vi "Post-Install Custom Action.vi"(10 "Variant":variant) -> (0 "error out":errorcluster)   [LabVIEW 2013]
uses:
  <vilib>/Utility/traverseref.llb/TRef TravTarget.ctl
  <vilib>/Utility/traverseref.llb/VI Scripting - Traverse.lvlib
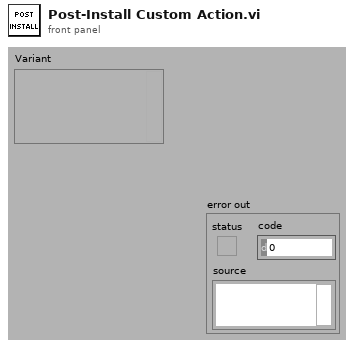
[diagram p1: front panel]
types:
  T1 = typedef "TRef TravTarget.ctl" = enum16{"FP", "BD", "Other"}
  T2 = enum32{"invalid VI type", "Standard VI", "Control VI", "Global VI", "Polymorphic VI", "Configuration VI", "SubSystem", "Facade VI", "Method VI", "Statechart Diagram VI"}
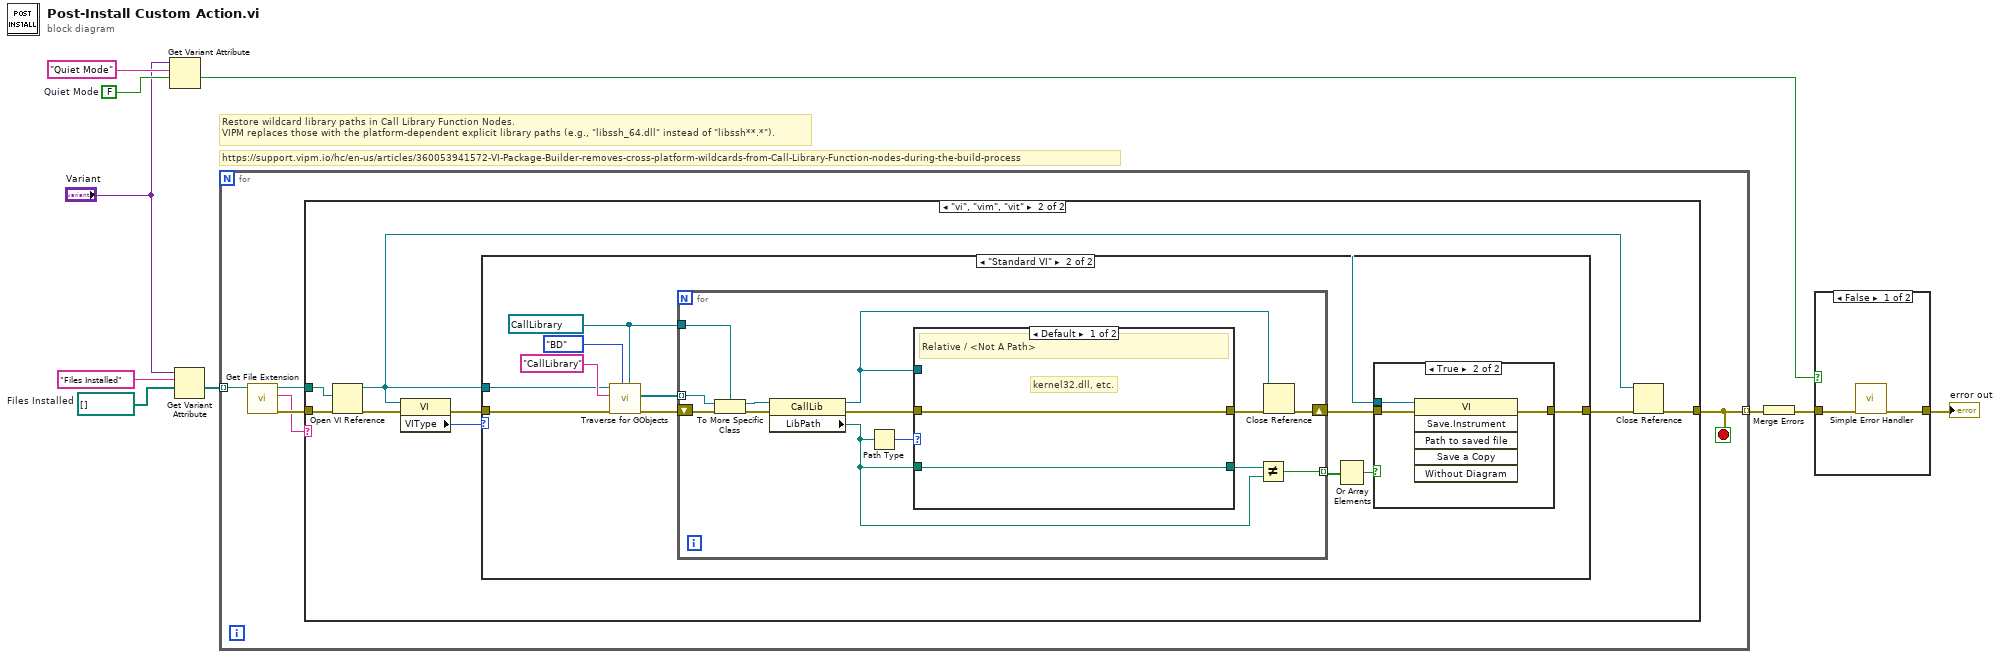
[diagram p0: block diagram]
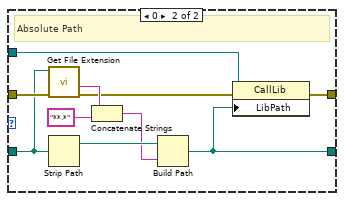
[diagram p6: hidden frame]
diagram:
  w5 = FALSE  # Quiet Mode
  w9 = path[] []  # Files Installed
  # "Restore wildcard library paths in Call Library Function Nodes.\nVIPM replaces those with the platform-dependent explicit library paths (e.g., \"libssh_64.dll\" instead of \"libssh**.*\")."
  # "https://support.vipm.io/hc/en-us/articles/360053941572-VI-Package-Builder-removes-cross-platform-wildcards-from-Call-Library-Function-nodes-during-the-build-process"
  n1 = Get Variant Attribute(Variant="Variant", name="Quiet Mode", default value (empty Variant)=w5) -> (value=w1:bool)  [unwired: 1 in, 3 out]
  n2 = Get Variant Attribute(Variant="Variant", name="Files Installed", default value (empty Variant)=w9) -> (value=w8:path[])  [unwired: 1 in, 3 out]
  n3 = for {
    tunnel: w8 -> [w15] mode=indexing
    tunnel: [w11] -> w7 mode=indexing
    stop <- w11 stop-if-true
    n4 = call <vilib>:"Get File Extension.vi"("file"=w15) -> ("error out"=w13:errorcluster, "lowercase file extension"=w12:string, "dup file"=w14:path)  [unwired: 7 in, 1 out]
    n5 = case shown="\"vi\", \"vim\", \"vit\"" w12 {
      tunnel: w14 -> [_ w24]
      tunnel: [w16 w22] -> w11
      tunnel: w13 -> [w16 w21]
      frame Default {
      }
      frame "vi", "vim", "vit" {
        n6 = Open VI Reference(vi path=w24, error in (no error)=w21) -> (vi reference=w18:refnum<vi>, error out=w20:errorcluster)  [unwired: 4 in]
        n7 = property class="VI"(reference=w18, error in=w20) -> (error out=w19:errorcluster, "VIType"=w17:T2)  [unwired: 1 out]
        n8 = case shown="\"Standard VI\"" w17 {
          tunnel: [w25 w28] -> w23
          tunnel: w19 -> [w25 w27]
          tunnel: w18 -> [_ w26]
          frame Default {
            # "Polimorphic VIs, etc."
          }
          frame "Standard VI" {
            w32 = refnum<vi> refnum ("Other Refnum")
            n9 = call <vilib>:"Traverse for GObjects.vi"("Other Refnum"=w32, "Traverse Target"=TRef_TravTarget."BD", "error in (no error)"=w27, "Class Name"="CallLibrary", "VI Refnum"=w26) -> ("error out"=w33:errorcluster, "References"=w34:refnum<vi>[])  [unwired: 3 in, 2 out]
            n10 = for {
              tunnel: w34 -> [w51] mode=indexing
              shift-right: [w45] -> w29
              shift-left: w33 -> [w53]
              tunnel: w32 -> [w52]
              tunnel: [w41] -> w31 mode=indexing
              n11 = To More Specific Class(target class=w52, reference=w51, error in=w53) -> (specific class reference=w49:refnum<vi>, error out=w50:errorcluster)
              n12 = property class="CallLib"(reference=w49, error in=w50) -> (reference out=w44:refnum<vi>, error out=w46:errorcluster, "LibPath"=w42:path)
              n13 = Path Type(1:w42) -> (0:w48:i16)
              n14 = case shown="Default" w48 {
                tunnel: [w55 w58] -> w47
                tunnel: w46 -> [w55 w65]
                tunnel: w42 -> [w54 w64]
                tunnel: w44 -> [_ w57]
                tunnel: [w54 w56] -> w43
                frame Default {
                  # "kernel32.dll, etc."
                  # "Relative / <Not A Path>"
                }
                frame 0 {
                  # "Absolute Path"
                  n15 = call <vilib>:"Get File Extension.vi"("error in (no error)"=w65, "file"=w64) -> ("error out"=w59:errorcluster, "filename without extension"=w63:string)  [unwired: 6 in, 2 out]
                  n16 = Strip Path(path=w64) -> (stripped path=w62:path)  [unwired: 1 out]
                  n17 = Concatenate Strings(w63, "**.*" ("string")) -> (w60:string)
                  n18 = Build Path(base path=w62, name or relative path=w60) -> (appended path=w56:path)
                  n19 = property class="CallLib"(reference=w57, error in=w59, "LibPath"=w56) -> (error out=w58:errorcluster)  [unwired: 1 out]
                }
              }
              n20 = Not Equal?(x=w43, y=w42) -> (x != y?=w41:bool)
              n21 = Close Reference(reference=w44, error in (no error)=w47) -> (error out=w45:errorcluster)
            }
            n22 = Or Array Elements(Boolean array=w31) -> (logical OR=w30:bool)
            n23 = case shown="True" w30 {
              tunnel: w26 -> [_ w40]
              tunnel: w29 -> [w37 w39]
              tunnel: [w37 w38] -> w28
              frame False {
              }
              frame True {
                n24 = invoke class="VI" method="Save.Instrument"(reference=w40, error in=w39) -> (error out=w38:errorcluster)  [unwired: 4 in, 5 out]
              }
            }
          }
        }
        n25 = Close Reference(reference=w18, error in (no error)=w23) -> (error out=w22:errorcluster)
      }
    }
  }
  n26 = Merge Errors(w7) -> (w2:errorcluster)
  n27 = case shown="False" w1 {
    tunnel: [w66 w68] -> w3
    tunnel: w2 -> [w67 w68]
    frame False {
      n28 = call <vilib>:"Simple Error Handler.vi"("error in (no error)"=w67) -> ("error out"=w66:errorcluster)  [unwired: 4 in, 4 out]
    }
    frame True {
    }
  }
  "error out" <- w3
